vi "sincosSGL.vi"(5 "x":sgl caption="x (pi radians)") -> (6 "sinx":sgl, 8 "cosx":sgl)   [LabVIEW 2015]
doc: "x is in units of pi radians."
panel:
  out "LUT":sgl[](array[numeric])
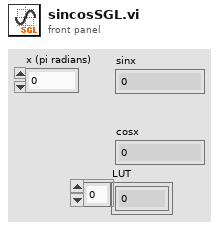
[diagram p1: front panel]
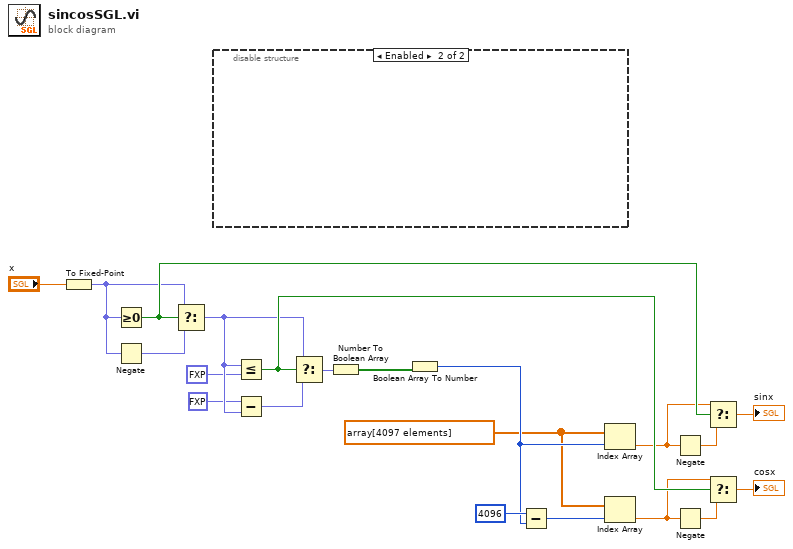
[diagram p0: block diagram]
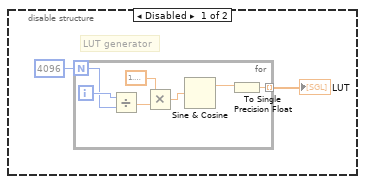
[diagram p2: hidden frame]
diagram:
  w1 = sgl[] array[4097 elements] ("LUT")
  n1 = To Fixed-Point(number="x") -> (fixed-point=w9:fxp<+/-,14,1>)  [unwired: 1 in]
  n2 = Greater Or Equal To 0?(x=w9) -> (x >= 0?=w18:bool)
  n3 = Negate(x=w9) -> (-x=w21:fxp<+/-,15,2>)
  n4 = Select(t=w9, s=w18, f=w21) -> (s? t:f=w11:fxp<+/-,15,2>)
  n5 = disable-structure shown="Enabled" {
    frame Disabled {
      # "LUT generator"
      n6 = for {
        N: 4096 -> [w29]
        tunnel: [w24] -> w22 mode=indexing
        i -> [w30]
        n7 = Divide(x=w30, y=w29) -> (x/y=w28:dbl)
        n8 = Multiply(x=1.5707963267948966, y=w28) -> (x*y=w26:dbl)
        n9 = Sine & Cosine(0:w26) -> (1:w25:dbl)  [unwired: 1 out]
        n10 = To Single Precision Float(number=w25) -> (single precision float=w24:sgl)
      }
      "LUT" <- w22
    }
    frame Enabled {
    }
  }
  n11 = Less Or Equal?(x=w11, y=fxp<+/-,14,2> 0.5) -> (x <= y?=w16:bool)
  n12 = Subtract(x=fxp<+/-,14,2> 1.0, y=w11) -> (x-y=w17:fxp<+/-,16,3>)
  n13 = Select(t=w11, s=w16, f=w17) -> (s? t:f=w6:fxp<+/-,16,3>)
  n14 = Number To Boolean Array(number=w6) -> (Boolean array=w5:bool[])
  n15 = Boolean Array To Number(Boolean array=w5) -> (number=w3:u16)
  n16 = Subtract(x=u16 4096, y=w3) -> (x-y=w2:u16)
  n17 = Index Array(array=w1, index=w3) -> (element=w13:sgl)
  n18 = Index Array(array=w1, index=w2) -> (element=w12:sgl)
  n19 = Negate(x=w13) -> (-x=w20:sgl)
  n20 = Negate(x=w12) -> (-x=w15:sgl)
  n21 = Select(t=w13, s=w18, f=w20) -> (s? t:f=→"sinx":sgl)
  n22 = Select(t=w12, s=w16, f=w15) -> (s? t:f=→"cosx":sgl)
